vi "checkinterference.vi"(9 "?":u8[][](array[numeric]), 11 "piece":u8[][](array[numeric])) -> (3 "?":bool)   [LabVIEW 2018]
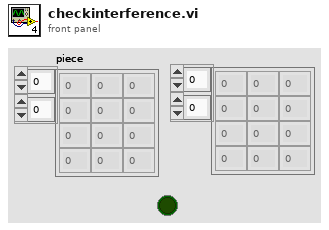
[diagram p1: front panel]
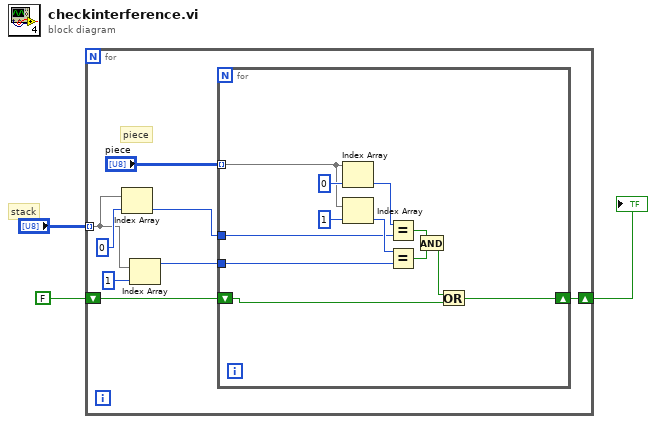
[diagram p0: block diagram]
diagram:
  # "stack"
  n1 = for {
    tunnel: "?" -> [w9] mode=indexing
    shift-right: [w4] -> w3
    shift-left: FALSE -> [w5]
    # "piece"
    n2 = Index Array(array=w9, index=0) -> (element=w7:u8)
    n3 = Index Array(array=w9, index=1) -> (element=w6:u8)
    n4 = for {
      tunnel: "piece" -> [w21] mode=indexing
      tunnel: w7 -> [w18]
      tunnel: w6 -> [w17]
      shift-right: [w13] -> w4
      shift-left: w5 -> [w14]
      n5 = Index Array(array=w21, index=0) -> (element=w20:u8)
      n6 = Index Array(array=w21, index=1) -> (element=w19:u8)
      n7 = Equal?(x=w20, y=w18) -> (x = y?=w16:bool)
      n8 = Equal?(x=w19, y=w17) -> (x = y?=w15:bool)
      n9 = And(x=w16, y=w15) -> (x .and. y?=w12:bool)
      n10 = Or(x=w12, y=w14) -> (x .or. y?=w13:bool)
    }
  }
  "?" <- w3
